vi "SimEx DC Motor Position Control with PID.vi"() -> ()   [LabVIEW 2020]
doc: "This example demonstrates how to use the PID function with Control Design and Simulation Module. Also demonstrates how to tune a PID Controller for position control of a DC Motor."
uses:
  <vilib>/Simulation/Scripting/Companion Diagram/SimConfigNode/SimParams.ctl
  <vilib>/Simulation/Scripting/Companion Diagram/SimConfigNode/_simSolvers.ctl
  <vilib>/Simulation/Implementation/Shared/SIMSCR Execution Mode.ctl
  <vilib>/Platform/TimedLoop/XDataNode/timing_clust.ctl
  <vilib>/Platform/TimedLoop/XDataNode/nitl_modes.ctl
  <vilib>/Platform/TimedLoop/XDataNode/wakeup.ctl
  <vilib>/Simulation/Param Hierarchy/Typedefs/SIMPH Param Control Actions.ctl
  <vilib>/Simulation/Implementation/Shared/SIM limit type.ctl
  <vilib>/Simulation/Scripting/Editor Utilities/SIM subVI tag data.ctl
  <vilib>/Simulation/Scripting/Editor Utilities/SIM subVI execution type.ctl
  <vilib>/Simulation/Implementation/Shared/NILVSim_ParamChanged.vi
  <vilib>/Simulation/Implementation/Shared/NILVSim_FinishedLate.vi
  <vilib>/Simulation/Implementation/Shared/NILVSIM_BeginStep.vi
  <vilib>/Simulation/Utility/Implementation/SIM Halt.vi
  <vilib>/Simulation/DiscreteLinear/Implementation/NILVSim Discrete State Space Buffered.llb/SIM Discrete State Space Distributor (SISO).vi
  <vilib>/Simulation/ContinuousLinear/Implementation/NILVSim Integrator new.llb/SIM Integrator distributor (scalar).vi
  <vilib>/Simulation/ContinuousLinear/Implementation/NILVSim Integrator new.llb/SIM Integrator collector (scalar).vi
  <vilib>/Simulation/Implementation/Shared/SIM Fire Discrete SubVI.vi
  <vilib>/Simulation/DiscreteLinear/Implementation/NILVSim Discrete State Space Buffered.llb/SIM Discrete State Space Collector (SISO).vi
  <vilib>/Simulation/Implementation/Shared/NILVSim_Manager.vi
  <vilib>/Utility/error.llb/Clear Errors.vi
  <vilib>/Simulation/Implementation/Shared/NILVSim_FinalizeModel.vi
  <vilib>/Simulation/Implementation/Shared/SIM Fire Discrete SubVI (Core).vi
  <vilib>/Simulation/Implementation/Shared/SIM Unbundle Sim Info.vi
  <vilib>/Simulation/Implementation/Shared/SIMSH Read Queue.vi
  <vilib>/Simulation/Implementation/Shared/NILVSim_Initialize.vi
  <vilib>/addons/control/pid/pid.llb/PID.vi
  <vilib>/addons/control/pid/pid.llb/PID (DBL).vi
  <vilib>/Simulation/Utility/Implementation/NILVSim Get Time and IsAcceptedStep.vi
  <vilib>/Simulation/Implementation/Shared/NILVSim_GetModelError.vi
  <vilib>/Simulation/Implementation/Shared/SIM Bundle Sim Info.vi
  <vilib>/Simulation/Scripting/Companion Diagram/SimConfigNode/SimDog.xnode
  <vilib>/Platform/TimedLoop/XDataNode/XDataNode.xnode
  <vilib>/Simulation/Implementation/XNodeFramework/SimXNode/SimX.xnode
  <vilib>/addons/control/pid/NI_PID_pid.lvlib
  <vilib>/Simulation/DiscreteLinear/Implementation/NILVSim Discrete State Space Buffered.llb/SIM Discrete State Space Buffered (SISO).vi
  <vilib>/Simulation/ContinuousLinear/Implementation/NILVSim Integrator new.llb/SIM Integrator (scalar).vi
  <vilib>/Platform/TimedLoop/XDataNode/XDNodeRunTimeDep.lvlib
  <vilib>/Simulation/Implementation/Shared/NI_SIM_Implementation.lvlib
panel:
  out "Time has Elapsed":bool
  out "Numeric":dbl
  out "Time":dbl
  in  "Td":dbl min=0.0 max=5.0 step=0.1 format="%#.4g"
  in  "Ti":dbl min=0.0 max=10.0 step=0.1 format="%#.4g"
  in  "Kc":dbl min=0.0 max=20.0 step=0.1
  in  "Reset control":bool
  in  "Disturbance":i32(slide) min=0 max=10 step=1 scale=0.0..10.0
  in  "Setpoint":dbl(slide) min=-3.14 max=3.14 step=0.1 scale=-3.14..3.14
  out "Voltage":dbl(slide) scale=-2.0..2.0
  out "Position":dbl(slide) scale=-3.0..3.0
  in  "Stop":bool
  out "Signal Response":cluster{"Setpoint:":dbl, "output y(k)":dbl}(graph)
  out "PV":dbl(knob) scale=-3.14..3.14
  # "Overview: This example demonstrates how to use the PID function with Control Design and Simulation Module. Also demonstrates how to tune a PID Controller for position control of a DC Motor.\nInstructions:\n1. Run the VI and verify how the PID Controller regulates the position.\n2. Try to add integral time  to the controller.\n3. Verify to add derivative time to the controller. Verify how the system behaves by changing setpoint and disturbance.\n4. Try the following gains for the PID with proportional gain as 8, integral time as 0.005 and derivative time as 0.001. Can you improve\nthis tuning?"
  # "Desired\nPosition\n(rad)"
  # "Position"
  # "Voltage"
  # "Position"
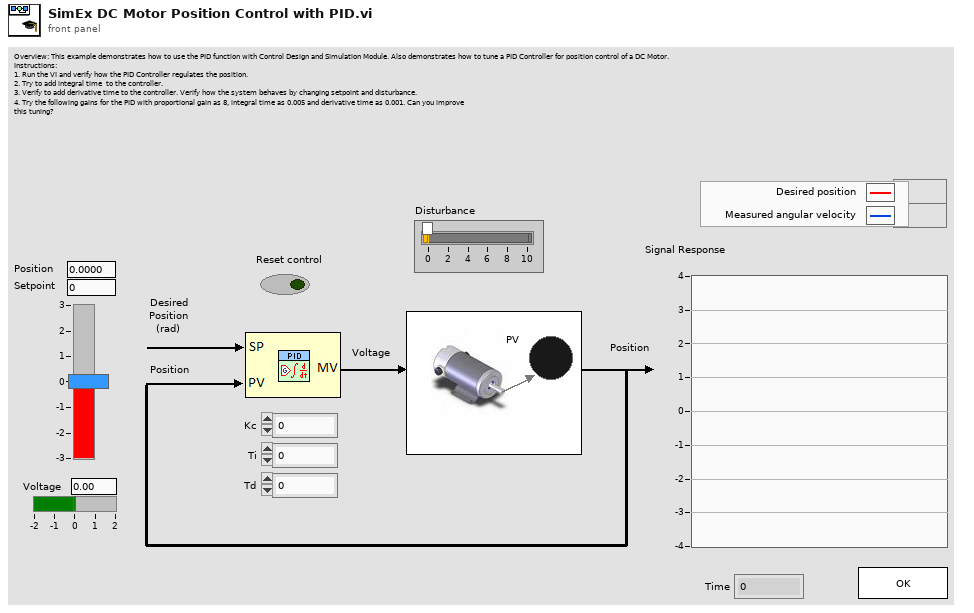
[diagram p1: front panel]
types:
  T1 = enum16{"Runge-Kutta 1 (Euler)", "Runge-Kutta 2", "Runge-Kutta 3", "Runge-Kutta 4", "Runge-Kutta 23 (variable)", "Runge-Kutta 45 (variable)", "BDF (variable)", "Adams-Moulton (variable)", "Rosenbrock (variable)", "Discrete States Only", "SDIRK 4 (variable)", "Radau 5 (variable)", "Radau 9 (variable)", "Radau 13 (variable)", "Radau [Variable Order] (variable)", "Gear's Method (variable)"}
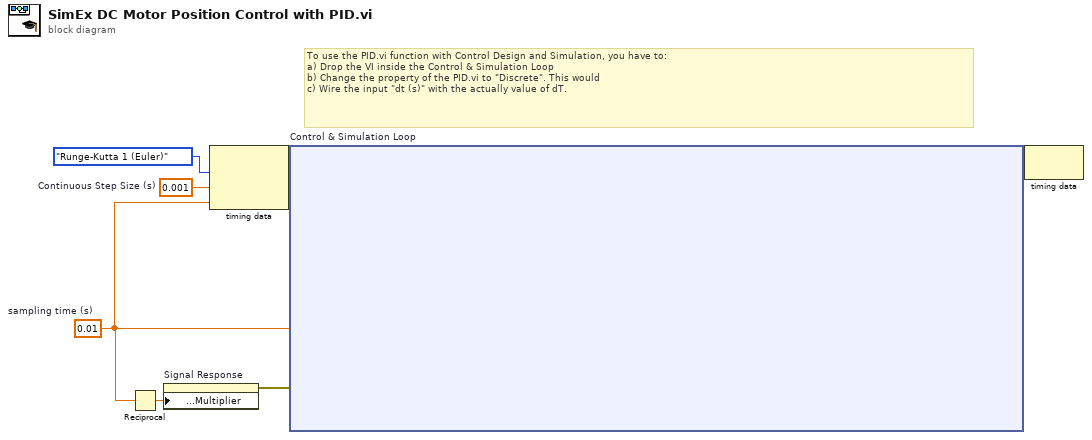
[diagram p0: block diagram]
diagram:
  w2 = 0.001  # Continuous Step Size (s)
  w3 = 0.01  # sampling time (s)
  # "To use the PID.vi function with Control Design and Simulation, you have to:\na) Drop the VI inside the Control & Simulation Loop\nb) Change the property of the PID.vi to \"Discrete\". This would\nc) Wire the input \"dt (s)\" with the actually value of dT."
  n1 = Reciprocal(x=w3) -> (1/x=w4:dbl)
  n2 = property on="Signal Response" class="WFChart (strict)"("X Scale.Offset and Multiplier:Multiplier"=w4) -> (error out=w7:errorcluster)  [unwired: 2 in, 1 out]
  n3 = node-c288(T1."Runge-Kutta 1 (Euler)" ("ODE Solver"), w2, w3) -> (w6:variant)
  n4 = node-c254 "Control & Simulation Loop"(w7, w6, w3) -> (w5:variant)
  n5 = node-c288(w5) -> ()  [unwired: 1 out]
